vi "Keyboard Packet.vi"() -> ()   [LabVIEW 2017]
uses:
  Robot Global Data.vi
  Common Code/Keyboard Packet.ctl
panel:
  in  "connection ID":refnum<k16>
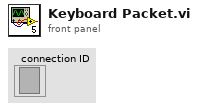
[diagram p1: front panel]
types:
  T1 = typedef "Keyboard Packet.ctl" = cluster{"keys pressed":enum16{"0", "1", "2", "3", "4", "5", "6", "7", "8", "9", "A", "B", "C", "D", "E", "F", "G", "H", "I", "J", "K", "L", "M", "N", "O", "P", "Q", "R", "S", "T", "U", "V", "W", "X", "Y", "Z", "F1", "F2", "F3", "F4", "F5", "F6", "F7", "F8", "F9", "F10", "F11", "F12", "F13", "F14", "F15", "ADD", "BACK", "BACKSLASH", "CAPITAL", "COMMA", "DECIMAL", "DELETE", "DIVIDE", "DOWN", "END", "EQUALS", "ESCAPE", "GRAVE (`)", "HOME", "INSERT", "LBRACKET", "LCONTROL", "LEFT", "L ALT", "LSHIFT", "LWIN", "MINUS", "MULTIPLY", "NEXT", "NUMLOCK", "NUMPAD_0", "NUMPAD_1", "NUMPAD_2", "NUMPAD_3", "NUMPAD_4", "NUMPAD_5", "NUMPAD_6", "NUMPAD_7", "NUMPAD_8", "NUMPAD_9", "PAUSE", "PERIOD", "PRIOR (PG UP)", "RBRACKET", "RCONTROL", "RETURN", "RIGHT", "R ALT", "RSHIFT", "RWIN", "SCROLL", "SEMICOLON", "SLASH", "SPACE", "SUBTRACT", "TAB", "UP", "ENTER (num pad)", "' (quote)"}[]}
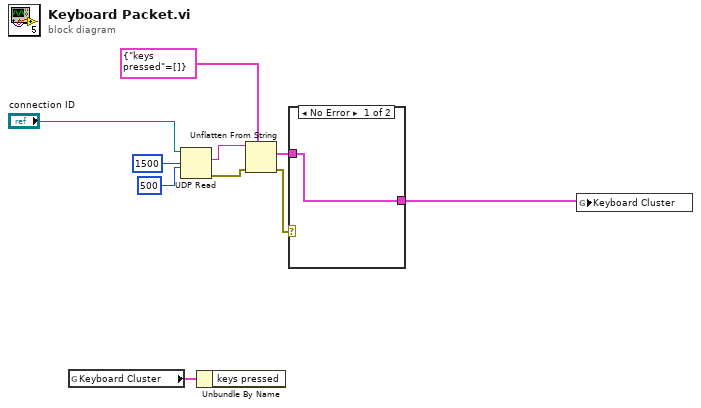
[diagram p0: block diagram]
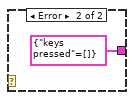
[diagram p2: hidden frame]
diagram:
  n1 = global read "Robot Global Data.vi" "Keyboard Cluster"() -> (w2:T1)
  n2 = UDP Read(connection ID="connection ID", max size (548)=1500, timeout ms (25000)=500) -> (data out=w8:string, error out=w6:errorcluster)  [unwired: 1 in, 3 out]
  n3 = Unbundle By Name(w2) -> ()  [unwired: 1 out]
  n4 = Unflatten From String(type=T1 {"keys pressed"=[]} ("Keyboard Cluster"), binary string=w8, error in (no error)=w6) -> (value=w7:T1, error out=w5:errorcluster)  [unwired: 2 in, 1 out]
  n5 = case shown="No Error" w5 {
    tunnel: w7 -> [w11 _]
    tunnel: [w11 T1 {"keys pressed"=[]} ("Keyboard Cluster")] -> w4
    frame No Error {
    }
    frame Error {
    }
  }
  n6 = global write "Robot Global Data.vi" "Keyboard Cluster"(w4) -> ()
